vi "PLC.ReasemblyDone.vi"(8 "error in":errorcluster, 10 "confirmed":bool=TRUE, 11 "Data_in":T1={"Status"={"Idx"=0, "ConnRef"=0, "State"=enum."Off", "LiveBitTimer"=timestamp(0 s since 1904-01-01)}, "Sets"={"Enable"=FALSE, "IP"="", "Rack"=0, "Slot"=0, "LifeBitTimer_s"=0.0, "DataBlockAddr_PCStatus"=0, "DataBlockAddr_PLCStatus"=1, "DataBlockAddr_PLCNewData"=[], "DataBlockSize_PLCNewData"=[], "DataBlockAddr_PLCChangeOver"=[], "DataBlockSize_PLCChangeOver"=[], "DataBlockAddr_PCChangeOver"=[], "DataBlockAddr_PLCCheckStatus"=[], "DataBlockSize_PLCCheckStatus"=[], "DataBlockAddr_PCCheckStatus"=[]}, "PCstatus"={"General"={"LifeBit"=FALSE, "DbRun"=FALSE}, "Stations"=[]}, "PLCstatus"={"General"={"LifeBit"=FALSE}, "Stations"=[]}}) -> (0 "error out":errorcluster, 2 "PlcConfirmation":T11, 3 "Data out":T1={"Status"={"Idx"=0, "ConnRef"=0, "State"=enum."Off", "LiveBitTimer"=timestamp(0 s since 1904-01-01)}, "Sets"={"Enable"=FALSE, "IP"="", "Rack"=0, "Slot"=0, "LifeBitTimer_s"=0.0, "DataBlockAddr_PCStatus"=0, "DataBlockAddr_PLCStatus"=1, "DataBlockAddr_PLCNewData"=[], "DataBlockSize_PLCNewData"=[], "DataBlockAddr_PLCChangeOver"=[], "DataBlockSize_PLCChangeOver"=[], "DataBlockAddr_PCChangeOver"=[], "DataBlockAddr_PLCCheckStatus"=[], "DataBlockSize_PLCCheckStatus"=[], "DataBlockAddr_PCCheckStatus"=[]}, "PCstatus"={"General"={"LifeBit"=FALSE, "DbRun"=FALSE}, "Stations"=[]}, "PLCstatus"={"General"={"LifeBit"=FALSE}, "Stations"=[]}})   [LabVIEW 2016]
uses:
  PLC.Data.ctl
  PLC.Data.Status.ctl
  PLC.State.ctl
  PLC.Data.Sets.ctl
  LowLevel/PLC.DataBlock.PCstatus.ctl
  LowLevel/PLC.DataBlock.PCstatus.General.ctl
  LowLevel/PLC.DataBlock.PCstatus.Station.ctl
  LowLevel/PLC.DataBlock.PLCstatus.ctl
  LowLevel/PLC.DataBlock.PLCstatus.General.ctl
  LowLevel/PLC.DataBlock.PLCstatus.Station.ctl
  PLC.CheckStatusReassembly.ctl
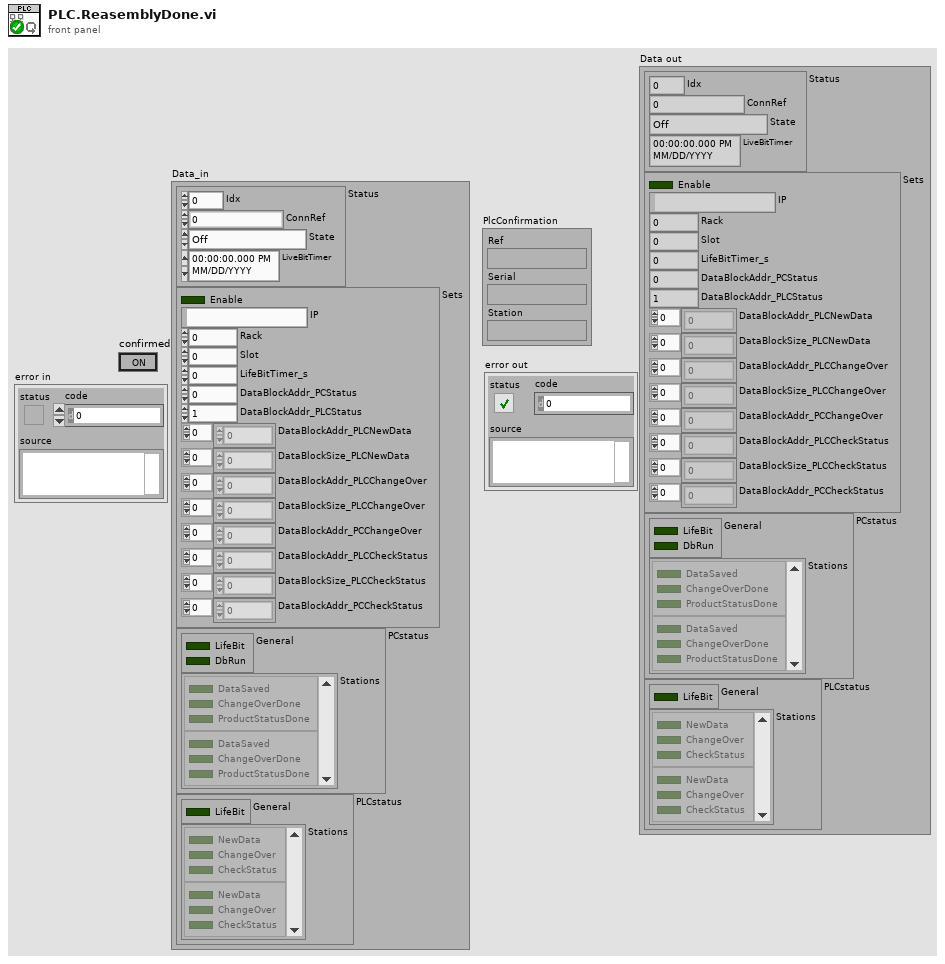
[diagram p1: front panel]
types:
  T1 = typedef "PLC.Data.ctl" = cluster{"Status":T2, "Sets":T4, "PCstatus":T5, "PLCstatus":T8}
  T2 = typedef "PLC.Data.Status.ctl" = cluster{"Idx":i32, "ConnRef":u64, "State":T3, "LiveBitTimer":timestamp}
  T3 = typedef "PLC.State.ctl" = enum32{"Off", "Error", "Idle", "Run"}
  T4 = typedef "PLC.Data.Sets.ctl" = cluster{"Enable":bool, "IP":string, "Rack":i32, "Slot":i32, "LifeBitTimer_s":dbl, "DataBlockAddr_PCStatus":i32, "DataBlockAddr_PLCStatus":i32, "DataBlockAddr_PLCNewData":i32[], "DataBlockSize_PLCNewData":i32[], "DataBlockAddr_PLCChangeOver":i32[], "DataBlockSize_PLCChangeOver":i32[], "DataBlockAddr_PCChangeOver":i32[], "DataBlockAddr_PLCCheckStatus":i32[], "DataBlockSize_PLCCheckStatus":i32[], "DataBlockAddr_PCCheckStatus":i32[]}
  T5 = typedef "PLC.DataBlock.PCstatus.ctl" = cluster{"General":T6, "Stations":T7[]}
  T6 = typedef "PLC.DataBlock.PCstatus.General.ctl" = cluster{"LifeBit":bool, "DbRun":bool}
  T7 = typedef "PLC.DataBlock.PCstatus.Station.ctl" = cluster{"DataSaved":bool, "ChangeOverDone":bool, "ProductStatusDone":bool}
  T8 = typedef "PLC.DataBlock.PLCstatus.ctl" = cluster{"General":T9, "Stations":T10[]}
  T9 = typedef "PLC.DataBlock.PLCstatus.General.ctl" = cluster{"LifeBit":bool}
  T10 = typedef "PLC.DataBlock.PLCstatus.Station.ctl" = cluster{"NewData":bool, "ChangeOver":bool, "CheckStatus":bool}
  T11 = typedef "PLC.CheckStatusReassembly.ctl" = cluster{"Ref":string, "Serial":string, "Station":string}
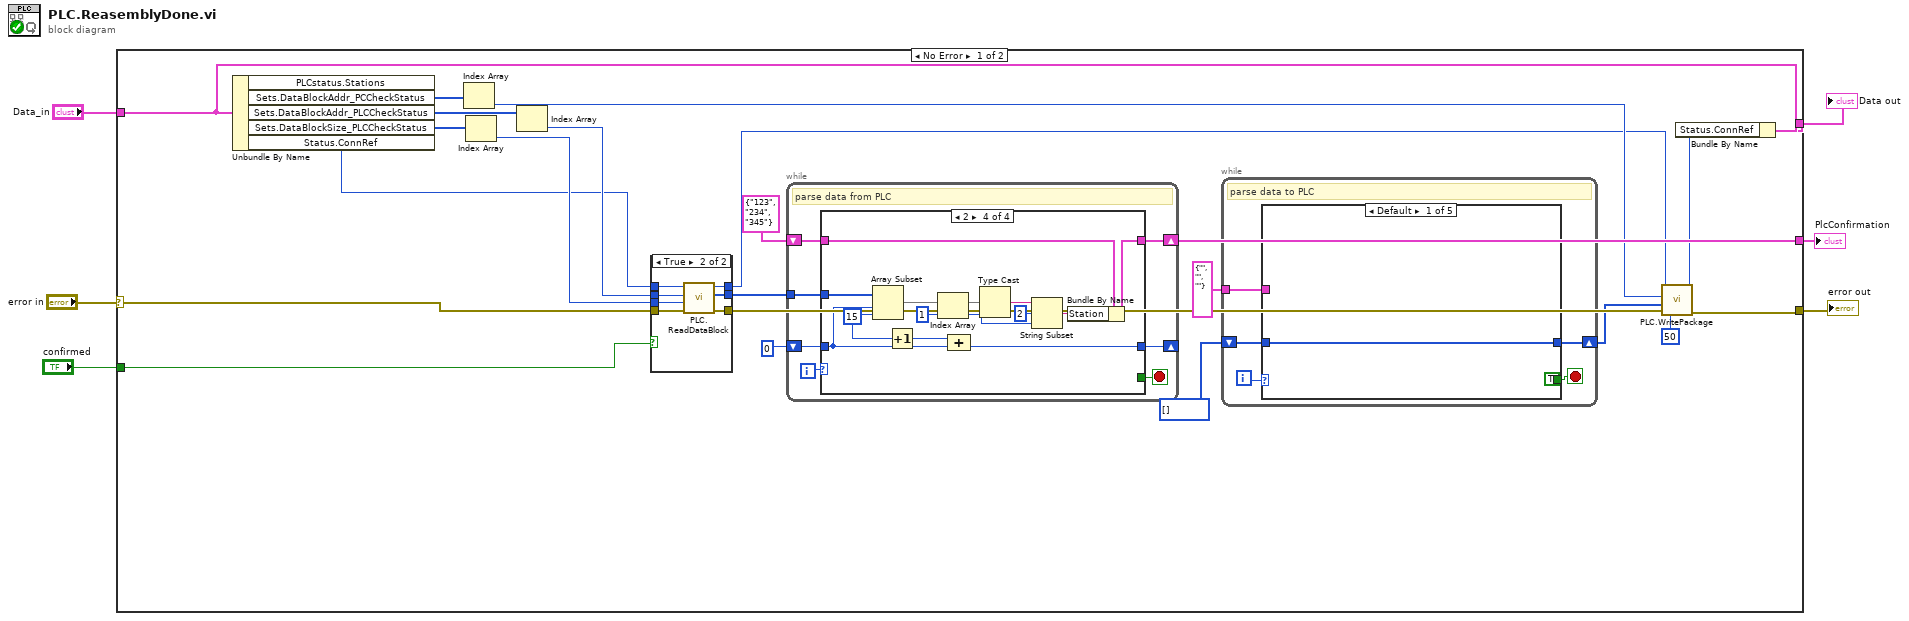
[diagram p0: block diagram]
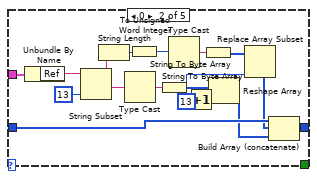
[diagram p3: hidden frame]
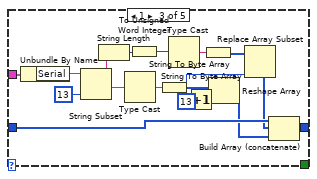
[diagram p4: hidden frame]
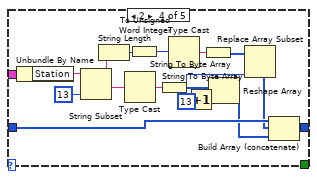
[diagram p5: hidden frame]
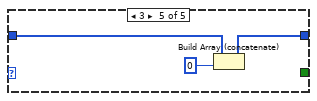
[diagram p6: hidden frame]
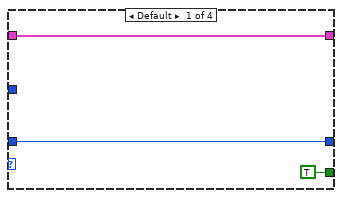
[diagram p7: hidden frame]
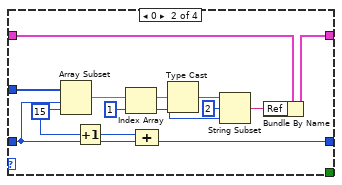
[diagram p8: hidden frame]
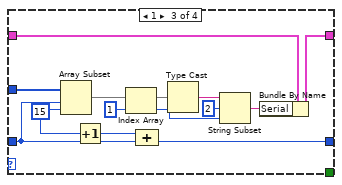
[diagram p9: hidden frame]
diagram:
  n1 = case shown="No Error" "error in" {
    selector: "error in" -> [w10 w147]
    tunnel: [w17 w147] -> w5
    tunnel: [w21 _] -> w4
    tunnel: "Data_in" -> [w20 w146]
    tunnel: [w19 w146] -> w2
    tunnel: "confirmed" -> [w7 _]
    frame No Error {
      n2 = Unbundle By Name(w20) -> ("Sets.DataBlockAddr_PCCheckStatus"=w29:i32[], "Sets.DataBlockAddr_PLCCheckStatus"=w28:i32[], "Sets.DataBlockSize_PLCCheckStatus"=w26:i32[], "Status.ConnRef"=w8:u64)  [unwired: 1 out]
      n3 = Index Array(array=w29) -> (element=w16:i32)  [unwired: 1 in]
      n4 = Index Array(array=w26) -> (element=w25:i32)  [unwired: 1 in]
      n5 = Index Array(array=w28) -> (element=w27:i32)  [unwired: 1 in]
      n6 = case shown="True" w7 {
        tunnel: w27 -> [_ w38]
        tunnel: w25 -> [_ w37]
        tunnel: [_ w36] -> w23
        tunnel: [w30 w35] -> w18
        tunnel: w10 -> [w30 w34]
        tunnel: [w31 w33] -> w9
        tunnel: w8 -> [w31 w32]
        frame False {
        }
        frame True {
          n7 = call "PLC.ReadDataBlock.vi"("error in (no error)"=w34, "Amount (1)"=w37, "Block"=w38, "Ref"=w32) -> ("error out"=w35:errorcluster, "data out"=w36:u8[], "ref out"=w33:u64)  [unwired: 5 in]
        }
      }
      n8 = while {
        tunnel: w23 -> [w98]
        shift-right: [w101] -> _
        shift-left: 0 -> [w102]
        shift-right: [w100] -> w21
        shift-left: T11 {"Ref"="123", "Serial"="234", "Station"="345"} ("Reasembly data 2") -> [w99]
        i -> [w103]
        stop <- w97 stop-if-true
        # "parse data from PLC"
        n9 = case shown="2" w103 {
          tunnel: w102 -> [w105 w110 w123 w136]
          tunnel: [w105 w109 w122 w135] -> w101
          tunnel: [w106 w119 w132 w145] -> w100
          tunnel: w99 -> [w106 w118 w131 w144]
          tunnel: w98 -> [_ w113 w126 w139]
          tunnel: [TRUE _ _ _] -> w97
          frame Default {
          }
          frame 0 {
            w111 = 15 ("length")
            n10 = Array Subset(array=w113, index=w110, length=w111) -> (w115:u8[])
            n11 = Increment(x=w111) -> (x+1=w107:i32)
            n12 = Index Array(array=w115, index=1) -> (element=w108:u8)
            n13 = Compound Arithmetic op=ADD(w107, w110) -> (w109:i32)
            n14 = Type Cast(x=w115) -> (*(type *) &x=w114:string)  [unwired: 1 in]
            n15 = String Subset(string=w114, offset (0)=2, length (rest)=w108) -> (substring=w112:string)
            n16 = Bundle By Name(cluster=w118, "Ref"=w112) -> (w119:T11)
          }
          frame 1 {
            w124 = 15 ("length")
            n17 = Array Subset(array=w126, index=w123, length=w124) -> (w128:u8[])
            n18 = Increment(x=w124) -> (x+1=w120:i32)
            n19 = Index Array(array=w128, index=1) -> (element=w121:u8)
            n20 = Compound Arithmetic op=ADD(w120, w123) -> (w122:i32)
            n21 = Type Cast(x=w128) -> (*(type *) &x=w127:string)  [unwired: 1 in]
            n22 = String Subset(string=w127, offset (0)=2, length (rest)=w121) -> (substring=w125:string)
            n23 = Bundle By Name(cluster=w131, "Serial"=w125) -> (w132:T11)
          }
          frame 2 {
            w137 = 15 ("length")
            n24 = Array Subset(array=w139, index=w136, length=w137) -> (w141:u8[])
            n25 = Increment(x=w137) -> (x+1=w133:i32)
            n26 = Index Array(array=w141, index=1) -> (element=w134:u8)
            n27 = Compound Arithmetic op=ADD(w133, w136) -> (w135:i32)
            n28 = Type Cast(x=w141) -> (*(type *) &x=w140:string)  [unwired: 1 in]
            n29 = String Subset(string=w140, offset (0)=2, length (rest)=w134) -> (substring=w138:string)
            n30 = Bundle By Name(cluster=w144, "Station"=w138) -> (w145:T11)
          }
        }
      }
      n31 = while {
        tunnel: T11 {"Ref"="", "Serial"="", "Station"=""} ("Reasembly data") -> [w42]
        shift-right: [w39] -> w14
        shift-left: u8[] [] -> [w40]
        i -> [w41]
        stop <- w43 stop-if-true
        # "parse data to PLC"
        n32 = case shown="Default" w41 {
          tunnel: w42 -> [_ w61 w77 w93 _]
          tunnel: [TRUE _ _ _ _] -> w43
          tunnel: [w44 w60 w76 w92 w95] -> w39
          tunnel: w40 -> [w44 w59 w75 w91 w96]
          frame Default {
          }
          frame 0 {
            w47 = 13
            n33 = Unbundle By Name(w61) -> ("Ref"=w57:string)
            n34 = String Subset(string=w57, length (rest)=13 ("length (rest)")) -> (substring=w53:string)  [unwired: 1 in]
            n35 = String Length(string=w53) -> (length=w58:i32)
            n36 = Type Cast(x=w53) -> (*(type *) &x=w54:string)  [unwired: 1 in]
            n37 = To Unsigned Word Integer(number=w58) -> (unsigned 16bit integer=w56:u16)
            n38 = String To Byte Array(string=w54) -> (unsigned byte array=w52:u8[])
            n39 = Type Cast(x=w56) -> (*(type *) &x=w55:string)  [unwired: 1 in]
            n40 = Increment(x=w47) -> (x+1=w46:i32)
            n41 = String To Byte Array(string=w55) -> (unsigned byte array=w49:u8[])
            n42 = Reshape Array(w52, w46) -> (w51:u8[])
            n43 = Replace Array Subset(array=w49, new element=w47) -> (w48:u8[])  [unwired: 1 in]
            n44 = Build Array (concatenate)(w59, w48, w51) -> (w60:i32[])
          }
          frame 1 {
            w63 = 13
            n45 = Unbundle By Name(w77) -> ("Serial"=w73:string)
            n46 = String Subset(string=w73, length (rest)=13 ("length (rest)")) -> (substring=w69:string)  [unwired: 1 in]
            n47 = String Length(string=w69) -> (length=w74:i32)
            n48 = Type Cast(x=w69) -> (*(type *) &x=w70:string)  [unwired: 1 in]
            n49 = To Unsigned Word Integer(number=w74) -> (unsigned 16bit integer=w72:u16)
            n50 = String To Byte Array(string=w70) -> (unsigned byte array=w68:u8[])
            n51 = Type Cast(x=w72) -> (*(type *) &x=w71:string)  [unwired: 1 in]
            n52 = Increment(x=w63) -> (x+1=w62:i32)
            n53 = String To Byte Array(string=w71) -> (unsigned byte array=w65:u8[])
            n54 = Reshape Array(w68, w62) -> (w67:u8[])
            n55 = Replace Array Subset(array=w65, new element=w63) -> (w64:u8[])  [unwired: 1 in]
            n56 = Build Array (concatenate)(w75, w64, w67) -> (w76:i32[])
          }
          frame 2 {
            w79 = 13
            n57 = Unbundle By Name(w93) -> ("Station"=w89:string)
            n58 = String Subset(string=w89, length (rest)=13 ("length (rest)")) -> (substring=w85:string)  [unwired: 1 in]
            n59 = String Length(string=w85) -> (length=w90:i32)
            n60 = Type Cast(x=w85) -> (*(type *) &x=w86:string)  [unwired: 1 in]
            n61 = To Unsigned Word Integer(number=w90) -> (unsigned 16bit integer=w88:u16)
            n62 = String To Byte Array(string=w86) -> (unsigned byte array=w84:u8[])
            n63 = Type Cast(x=w88) -> (*(type *) &x=w87:string)  [unwired: 1 in]
            n64 = Increment(x=w79) -> (x+1=w78:i32)
            n65 = String To Byte Array(string=w87) -> (unsigned byte array=w81:u8[])
            n66 = Reshape Array(w84, w78) -> (w83:u8[])
            n67 = Replace Array Subset(array=w81, new element=w79) -> (w80:u8[])  [unwired: 1 in]
            n68 = Build Array (concatenate)(w91, w80, w83) -> (w92:i32[])
          }
          frame 3 {
            n69 = Build Array (concatenate)(w96, 0) -> (w95:i32[])
          }
        }
      }
      n70 = call "PLC.WritePackage.vi"("max package size  (0: full)"=50, "error in (no error)"=w18, "data"=w14, "addr"=w16, "Ref in"=w9) -> ("error out"=w17:errorcluster, "Ref out"=w15:u64)  [unwired: 5 in]
      n71 = Bundle By Name(cluster=w20, "Status.ConnRef"=w15) -> (w19:T1)
    }
    frame Error {
    }
  }
  "error out" <- w5
  "Data out" <- w2
  "PlcConfirmation" <- w4
